vi "Unpad Time Series Data.vi"(11 "Padded Time Series Data":dbl[][](array[numeric])) -> (3 "Unpadded Time Series Data":dbl[][](array[numeric]))   [LabVIEW 2013, in "Data Log Fetcher.lvlib"]
uses:
  Data Log Fetcher.lvlib
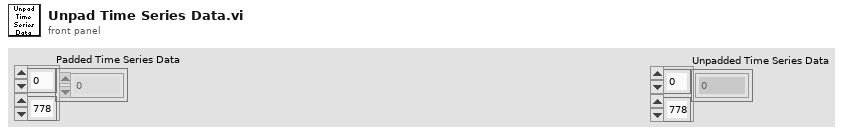
[diagram p1: front panel]
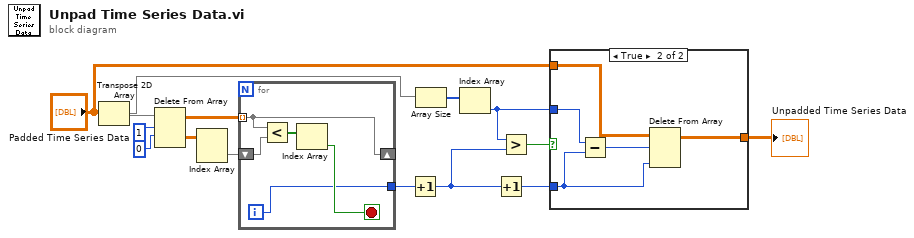
[diagram p0: block diagram]
diagram:
  n1 = Transpose 2D Array(2D array="Padded Time Series Data") -> (transposed array=w7:dbl[][])
  n2 = Delete From Array(array=w7, length=1, index (row)=0 ("disabled index (col)")) -> (deleted portion=w11:dbl[][], array with subset deleted=w12:dbl[][])  [unwired: 1 in]
  n3 = Index Array(array=w11) -> (element=w10:dbl[])  [unwired: 2 in]
  n4 = for {
    tunnel: w12 -> [w16] mode=indexing
    shift-right: [w16] -> _
    shift-left: w10 -> [w19]
    tunnel: [w15] -> w9
    i -> [w15]
    stop <- w17 stop-if-true
    n5 = Less?(x=w16, y=w19) -> (x < y?=w18:bool[])
    n6 = Index Array(array=w18) -> (element=w17:bool)  [unwired: 1 in]
  }
  n7 = Increment(x=w9) -> (x+1=w2:i32)
  n8 = Array Size(array=w7) -> (size(s)=w8:i32[])
  n9 = Index Array(array=w8) -> (element=w4:i32)  [unwired: 1 in]
  n10 = Increment(x=w2) -> (x+1=w1:i32)
  n11 = Greater?(x=w4, y=w2) -> (0:w6:bool)
  n12 = case shown="True" w6 {
    tunnel: w1 -> [_ w22]
    tunnel: "Padded Time Series Data" -> [w20 w25]
    tunnel: w4 -> [_ w24]
    tunnel: [w20 w21] -> w3
    frame False {
    }
    frame True {
      n13 = Subtract(x=w24, y=w22) -> (x-y=w23:i32)
      n14 = Delete From Array(array=w25, length=w23, index (col)=w22) -> (array with subset deleted=w21:dbl[][])  [unwired: 1 in, 1 out]
    }
  }
  "Unpadded Time Series Data" <- w3
